vi "Formic Princess.vi"(8 "error in (no error)":errorcluster, 11 "Mother in":refnum<class "Mother.lvclass">) -> (0 "error out":errorcluster, 3 "Mother out":refnum<class "Mother.lvclass">)   [LabVIEW 2014, in "Mother.lvclass"]
uses:
  Mother.lvclass
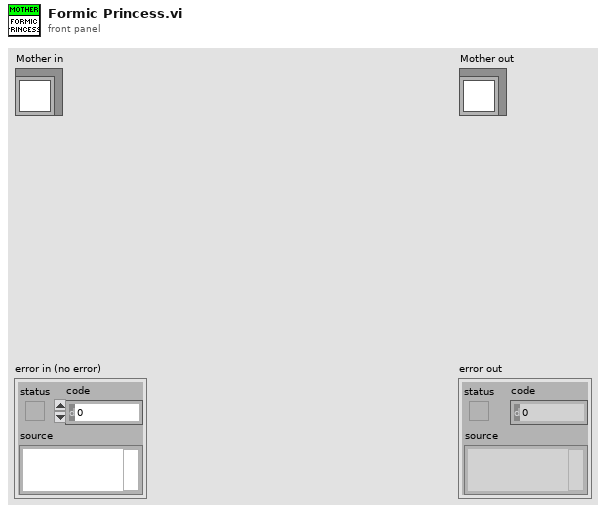
[diagram p1: front panel]
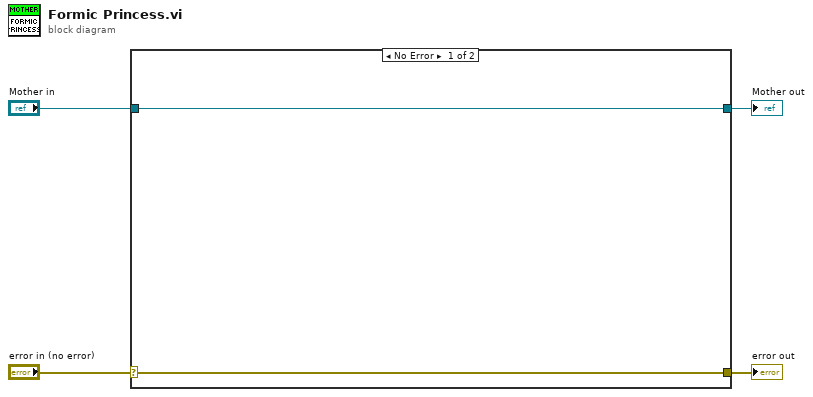
[diagram p0: block diagram]
diagram:
  n1 = case shown="No Error" "error in (no error)" {
    selector: "error in (no error)" -> [w5 w8]
    tunnel: [w5 w8] -> w3
    tunnel: [w6 w7] -> w1
    tunnel: "Mother in" -> [w6 w7]
    frame No Error {
    }
    frame Error {
    }
  }
  "error out" <- w3
  "Mother out" <- w1
